vi "restore_config.vi"(3 "Auto Load Default?":bool) -> ()   [LabVIEW 2012]
doc: "Restores the chirp pulse experiment settings from a config file."
uses:
  <vilib>/Utility/config.llb/Read Key (I32).vi
  global.vi
  <vilib>/Utility/config.llb/Read Key (Boolean).vi
  <vilib>/Utility/config.llb/Read Key (Double).vi
  <vilib>/Utility/config.llb/Read Key (String).vi
  <vilib>/Utility/config.llb/Read Key (Path).vi
  <vilib>/Utility/config.llb/NI_LVConfig.lvlib
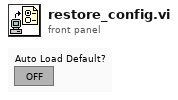
[diagram p1: front panel]
types:
  T1 = typedef "NI_LVConfig.lvlib/Config Data RefNum.ctl" = refnum<k1>
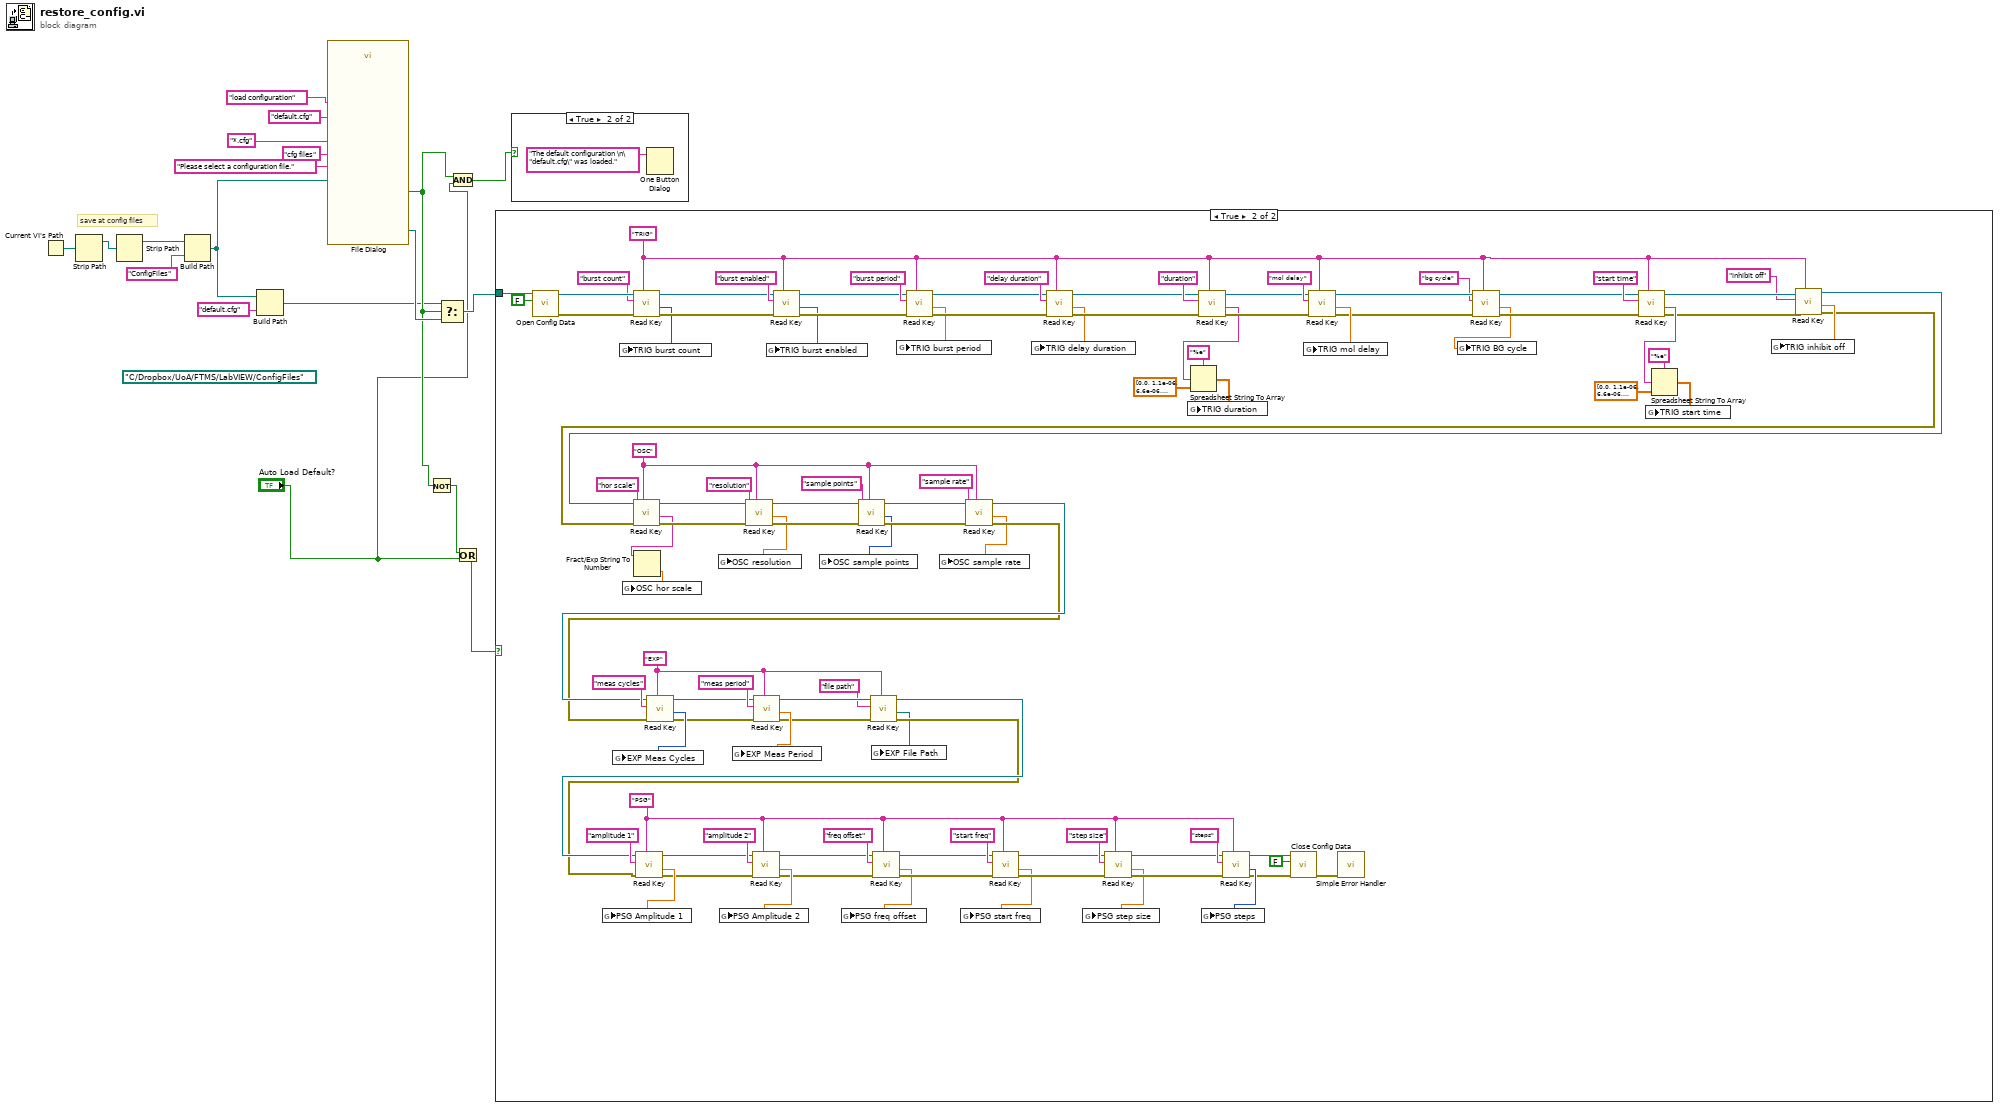
[diagram p0: block diagram]
diagram:
  (unwired) path "C:/Dropbox/UoA/FTMS/LabVIEW/ConfigFiles" ("t")
  # "save at config files"
  n1 = Current VI's Path() -> (path=w14:path)
  n2 = Strip Path(path=w14) -> (stripped path=w12:path)  [unwired: 1 out]
  n3 = Strip Path(path=w12) -> (stripped path=w11:path)  [unwired: 1 out]
  n4 = Build Path(base path=w11, name or relative path="ConfigFiles") -> (appended path=w3:path)
  n5 = Build Path(base path=w3, name or relative path="default.cfg") -> (appended path=w1:path)
  n6 = call "File Dialog"("start path"=w3, "prompt"="Please select a configuration file.", "button label"="load configuration", "default name"="default.cfg", "pattern (all files)"="*.cfg" ("default name"), "pattern label"="cfg files") -> ("selected path"=w10:path, "cancelled"=w5:bool)  [unwired: 6 in, 2 out]
  n7 = Not(x=w5) -> (.not. x?=w7:bool)
  n8 = Select(t=w1, s=w5, f=w10) -> (s? t:f=w9:path)
  n9 = And(x=w5, y="Auto Load Default?") -> (x .and. y?=w6:bool)
  n10 = Or(x=w7, y="Auto Load Default?") -> (x .or. y?=w8:bool)
  n11 = case shown="True" w8 {
    tunnel: w9 -> [_ w124]
    frame False {
    }
    frame True {
      w52 = "PSG"
      w22 = "EXP"
      w93 = "OSC"
      w27 = "TRIG"
      n12 = call <vilib>:"Open Config Data.vi"("create file if necessary (T)"=FALSE, "configuration file path"=w124) -> ("error out"=w122:errorcluster, "refnum"=w123:T1)  [unwired: 1 in, 7 out]
      n13 = call-poly <vilib>:"Read Key.vi"("section"=w27, "error in (no error)"=w122, "key"="burst count" ("Key 1"), "refnum"=w123) -> ("error out"=w111:errorcluster, "value"=w78:i32, "refnum out"=w115:T1)  [unwired: 4 in, 1 out]
      n14 = global write "global.vi" "TRIG burst count"(w78) -> ()
      n15 = call-poly <vilib>:"Read Key.vi"("section"=w27, "error in (no error)"=w111, "key"="burst enabled" ("Key 1"), "refnum"=w115) -> ("error out"=w110:errorcluster, "value"=w77:bool, "refnum out"=w114:T1)  [unwired: 4 in, 1 out]
      n16 = global write "global.vi" "TRIG burst enabled"(w77) -> ()
      n17 = call-poly <vilib>:"Read Key.vi"("section"=w27, "error in (no error)"=w110, "key"="burst period" ("Key 1"), "refnum"=w114) -> ("error out"=w109:errorcluster, "value"=w76:dbl, "refnum out"=w113:T1)  [unwired: 4 in, 1 out]
      n18 = global write "global.vi" "TRIG burst period"(w76) -> ()
      n19 = call-poly <vilib>:"Read Key.vi"("section"=w27, "error in (no error)"=w109, "key"="delay duration" ("Key 1"), "refnum"=w113) -> ("error out"=w108:errorcluster, "value"=w75:dbl, "refnum out"=w112:T1)  [unwired: 4 in, 1 out]
      n20 = global write "global.vi" "TRIG delay duration"(w75) -> ()
      n21 = call-poly <vilib>:"Read Key.vi"("section"=w27, "error in (no error)"=w108, "key"="duration" ("Key 1"), "refnum"=w112) -> ("error out"=w104:errorcluster, "value"=w72:string, "refnum out"=w105:T1)  [unwired: 4 in, 1 out]
      n22 = Spreadsheet String To Array(format string="%e", spreadsheet string=w72, array type (2D Dbl)=dbl[] [0.0, 1.1e-06, 6.6e-06, 6.4e-06] ("TRIG start time")) -> (array=w73:dbl[])  [unwired: 1 in]
      n23 = global write "global.vi" "TRIG duration"(w73) -> ()
      n24 = call-poly <vilib>:"Read Key.vi"("section"=w27, "error in (no error)"=w104, "key"="mol delay" ("Key 1"), "refnum"=w105) -> ("error out"=w37:errorcluster, "value"=w67:dbl, "refnum out"=w36:T1)  [unwired: 4 in, 1 out]
      n25 = global write "global.vi" "TRIG mol delay"(w67) -> ()
      n26 = call-poly <vilib>:"Read Key.vi"("section"=w27, "error in (no error)"=w37, "key"="bg cycle" ("Key 1"), "refnum"=w36) -> ("error out"=w38:errorcluster, "value"=w34:dbl, "refnum out"=w39:T1)  [unwired: 4 in, 1 out]
      n27 = global write "global.vi" "TRIG BG cycle"(w34) -> ()
      n28 = call-poly <vilib>:"Read Key.vi"("section"=w27, "error in (no error)"=w38, "key"="start time" ("Key 1"), "refnum"=w39) -> ("error out"=w32:errorcluster, "value"=w66:string, "refnum out"=w33:T1)  [unwired: 4 in, 1 out]
      n29 = Spreadsheet String To Array(format string="%e", spreadsheet string=w66, array type (2D Dbl)=dbl[] [0.0, 1.1e-06, 6.6e-06, 6.4e-06] ("TRIG start time")) -> (array=w69:dbl[])  [unwired: 1 in]
      n30 = global write "global.vi" "TRIG start time"(w69) -> ()
      n31 = call-poly <vilib>:"Read Key.vi"("section"=w27, "error in (no error)"=w32, "key"="inhibit off" ("Key 1"), "refnum"=w33) -> ("error out"=w28:errorcluster, "value"=w30:dbl, "refnum out"=w29:T1)  [unwired: 4 in, 1 out]
      n32 = call-poly <vilib>:"Read Key.vi"("section"=w93, "error in (no error)"=w28, "key"="hor scale" ("Key 1"), "refnum"=w29) -> ("error out"=w98:errorcluster, "value"=w45:string, "refnum out"=w100:T1)  [unwired: 4 in, 1 out]
      n33 = Fract/Exp String To Number(string=w45) -> (number=w44:dbl)  [unwired: 3 in, 1 out]
      n34 = global write "global.vi" "OSC hor scale"(w44) -> ()
      n35 = call-poly <vilib>:"Read Key.vi"("section"=w93, "error in (no error)"=w98, "key"="resolution" ("Key 1"), "refnum"=w100) -> ("error out"=w97:errorcluster, "value"=w65:dbl, "refnum out"=w99:T1)  [unwired: 4 in, 1 out]
      n36 = global write "global.vi" "OSC resolution"(w65) -> ()
      n37 = call-poly <vilib>:"Read Key.vi"("section"=w93, "error in (no error)"=w97, "key"="sample points" ("Key 1"), "refnum"=w99) -> ("error out"=w94:errorcluster, "value"=w64:i32, "refnum out"=w95:T1)  [unwired: 4 in, 1 out]
      n38 = global write "global.vi" "OSC sample points"(w64) -> ()
      n39 = call-poly <vilib>:"Read Key.vi"("section"=w93, "error in (no error)"=w94, "key"="sample rate" ("Key 1"), "refnum"=w95) -> ("error out"=w90:errorcluster, "value"=w63:dbl, "refnum out"=w91:T1)  [unwired: 4 in, 1 out]
      n40 = call-poly <vilib>:"Read Key.vi"("section"=w22, "error in (no error)"=w90, "key"="meas cycles" ("Key 1"), "refnum"=w91) -> ("error out"=w41:errorcluster, "value"=w62:i32, "refnum out"=w42:T1)  [unwired: 4 in, 1 out]
      n41 = global write "global.vi" "EXP Meas Cycles"(w62) -> ()
      n42 = call-poly <vilib>:"Read Key.vi"("section"=w22, "error in (no error)"=w41, "key"="meas period" ("Key 1"), "refnum"=w42) -> ("error out"=w25:errorcluster, "value"=w40:dbl, "refnum out"=w26:T1)  [unwired: 4 in, 1 out]
      n43 = global write "global.vi" "EXP Meas Period"(w40) -> ()
      n44 = call-poly <vilib>:"Read Key.vi"("section"=w22, "error in (no error)"=w25, "key"="file path", "refnum"=w26) -> ("error out"=w23:errorcluster, "value"=w20:path, "refnum out"=w24:T1)  [unwired: 4 in, 1 out]
      n45 = call-poly <vilib>:"Read Key.vi"("section"=w52, "error in (no error)"=w23, "key"="amplitude 1" ("Key 1"), "refnum"=w24) -> ("error out"=w47:errorcluster, "value"=w55:dbl, "refnum out"=w49:T1)  [unwired: 4 in, 1 out]
      n46 = global write "global.vi" "PSG Amplitude 1"(w55) -> ()
      n47 = call-poly <vilib>:"Read Key.vi"("section"=w52, "error in (no error)"=w47, "key"="amplitude 2" ("Key 1"), "refnum"=w49) -> ("error out"=w46:errorcluster, "value"=w53:dbl, "refnum out"=w48:T1)  [unwired: 4 in, 1 out]
      n48 = global write "global.vi" "PSG Amplitude 2"(w53) -> ()
      n49 = global write "global.vi" "EXP File Path"(w20) -> ()
      n50 = call-poly <vilib>:"Read Key.vi"("section"=w52, "error in (no error)"=w46, "key"="freq offset" ("Key 1"), "refnum"=w48) -> ("error out"=w84:errorcluster, "value"=w61:dbl, "refnum out"=w86:T1)  [unwired: 4 in, 1 out]
      n51 = global write "global.vi" "PSG freq offset"(w61) -> ()
      n52 = global write "global.vi" "OSC sample rate"(w63) -> ()
      n53 = call-poly <vilib>:"Read Key.vi"("section"=w52, "error in (no error)"=w84, "key"="start freq" ("Key 1"), "refnum"=w86) -> ("error out"=w83:errorcluster, "value"=w60:dbl, "refnum out"=w85:T1)  [unwired: 4 in, 1 out]
      n54 = global write "global.vi" "PSG start freq"(w60) -> ()
      n55 = call-poly <vilib>:"Read Key.vi"("section"=w52, "error in (no error)"=w83, "key"="step size" ("Key 1"), "refnum"=w85) -> ("error out"=w80:errorcluster, "value"=w59:dbl, "refnum out"=w81:T1)  [unwired: 4 in, 1 out]
      n56 = global write "global.vi" "PSG step size"(w59) -> ()
      n57 = call-poly <vilib>:"Read Key.vi"("section"=w52, "error in (no error)"=w80, "key"="steps" ("Key 1"), "refnum"=w81) -> ("error out"=w50:errorcluster, "value"=w58:i32, "refnum out"=w51:T1)  [unwired: 4 in, 1 out]
      n58 = global write "global.vi" "PSG steps"(w58) -> ()
      n59 = call <vilib>:"Close Config Data.vi"("error in (no error)"=w50, "write file if changed (T)"=FALSE, "refnum"=w51) -> ("error out"=w120:errorcluster)  [unwired: 8 out]
      n60 = call <vilib>:"Simple Error Handler.vi"("error in (no error)"=w120) -> ()  [unwired: 1 in, 8 out]
      n61 = global write "global.vi" "TRIG inhibit off"(w30) -> ()
    }
  }
  n62 = case shown="True" w6 {
    frame False {
    }
    frame True {
      n63 = One Button Dialog(message="The default configuration \n\"default.cfg\" was loaded.") -> ()  [unwired: 1 in, 1 out]
    }
  }
